vi "Breakdown Cluster.vi"(8 "error in (no error)":errorcluster, 10 "Cluster":variant) -> (0 "error out":errorcluster, 1 "values":variant[](array[variant]), 2 "tags":string[](array[string]))   [LabVIEW 2023, in "uData.lvlib" / "uData.lvclass"]
doc: "Use to break down the cluster elements into an array of tag labels and values. Nested clusters use a label[dot]sublabel notation."
uses:
  uData.lvclass
  <vilib>/Utility/error.llb/Trim Whitespace One-Sided.vi
  <vilib>/Utility/error.llb/Error Cluster From Error Code.vi
  <vilib>/ErrorRing/Error Ring.xnode
  <vilib>/Utility/Data Type/NI_Data Type.lvlib
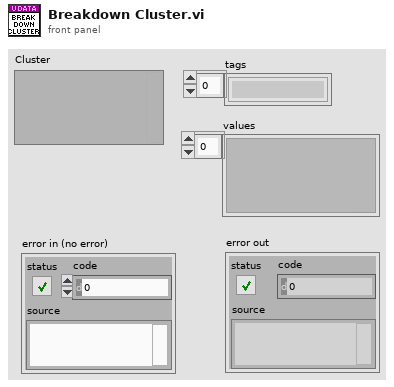
[diagram p1: front panel]
types:
  T1 = typedef "NI_Data Type.lvlib/Data Type.ctl" = enum8{"Invalid Type", "Void", "I8", "I16", "I32", "I64", "U8", "U16", "U32", "U64", "Single Float", "Double Float", "Extended Float", "Single Complex", "Double Complex", "Extended Complex", "Enum U8", "Enum U16", "Enum U32", "Enum U64", "Single Float With Unit", "Double Float With Unit", "Extended Float With Unit", "Single Complex with Unit", "Double Complex with Unit", "Extended Complex with Unit", "Boolean", "String", "Path", "Picture", "Tag", "Array", "Cluster", "Variant", "LV Variant", "Waveform", "Timestamp", "Digital Waveform", "Digital Data", "ExpressData", "Refnum", "External Data", "VI", "Poly VI", "LabVIEW Class Instance", "Fixed Point", "Set Collection", "Map Collection"}
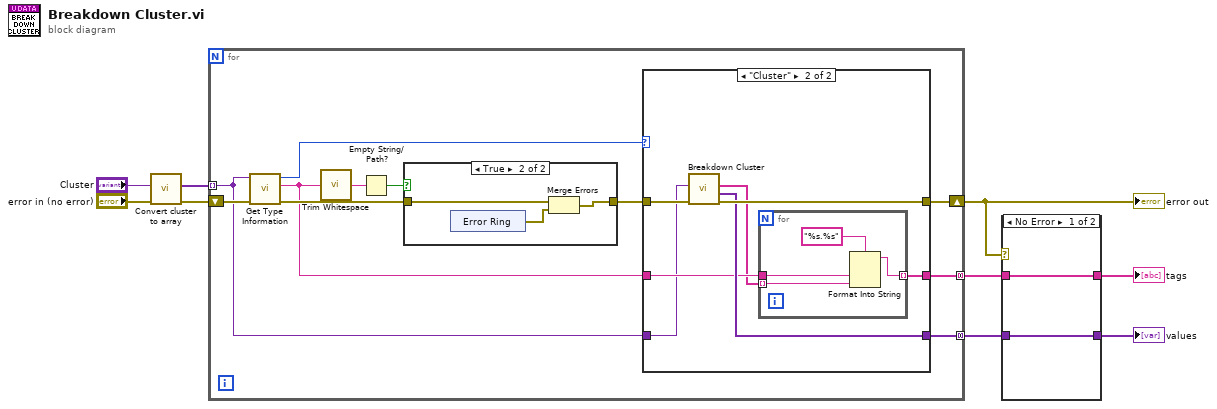
[diagram p0: block diagram]
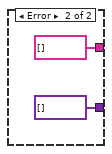
[diagram p2: hidden frame]
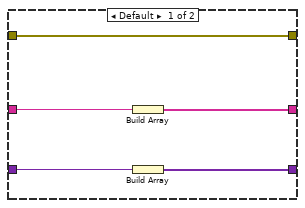
[diagram p4: hidden frame]
diagram:
  n1 = call "Convert cluster to array.vi"("error in (no error)"="error in (no error)", "cluster"="Cluster") -> ("error out"=w3:errorcluster, "array"=w2:variant[])  [unwired: 8 in]
  n2 = for {
    shift-right: [w18] -> w9
    shift-left: w3 -> [w20]
    tunnel: [w11] -> w7 mode=concatenating
    tunnel: w2 -> [w12] mode=indexing
    tunnel: [w10] -> w5 mode=concatenating
    n3 = call <vilib>:"Get Type Information.vi"("error in (no error)"=w20, "variant"=w12) -> ("error out"=w15:errorcluster, "name"=w13:string, "type"=w19:T1)  [unwired: 5 in, 2 out]
    n4 = call <vilib>:"Trim Whitespace.vi"("string"=w13) -> ("trimmed string"=w17:string)  [unwired: 1 in]
    n5 = Empty String/Path?(string/path=w17) -> (empty?=w16:bool)
    n6 = case shown="True" w16 {
      tunnel: w15 -> [w21 w24]
      tunnel: [w21 w23] -> w14
      frame False {
      }
      frame True {
        n7 = xnode "Error Ring"() -> ("error out"=w22:errorcluster)
        n8 = Merge Errors(w24, w22) -> (w23:errorcluster)
      }
    }
    n9 = case shown="\"Cluster\"" w19 {
      tunnel: [w34 w41] -> w18
      tunnel: w14 -> [w34 w40]
      tunnel: w13 -> [w33 w38]
      tunnel: w12 -> [w32 w35]
      tunnel: [w31 w36] -> w11
      tunnel: [w30 w39] -> w10
      frame Default {
        n10 = Build Array(w33) -> (w31:string[])
        n11 = Build Array(w32) -> (w30:variant[])
      }
      frame "Cluster" {
        n12 = call "Breakdown Cluster.vi"("error in (no error)"=w40, "Cluster"=w35) -> ("error out"=w41:errorcluster, "values"=w39:variant[], "tags"=w37:string[])  [unwired: 7 in]
        n13 = for {
          tunnel: w38 -> [w45]
          tunnel: w37 -> [w43] mode=indexing
          tunnel: [w42] -> w36 mode=indexing
          n14 = Format Into String(format string="%s.%s", w45, w43) -> (resulting string=w42:string)  [unwired: 2 in, 1 out]
        }
      }
    }
  }
  "error out" <- w9
  n15 = case shown="No Error" w9 {
    tunnel: [w47 string[] []] -> w8
    tunnel: w7 -> [w47 _]
    tunnel: [w46 variant[] []] -> w6
    tunnel: w5 -> [w46 _]
    frame No Error {
    }
    frame Error {
    }
  }
  "tags" <- w8
  "values" <- w6
